vi "Conv_Meters_Feet.vi"(10 "Meters":dbl) -> (2 "Feet":dbl)   [LabVIEW 2019, in "PathExecution_Library.lvlib"]
doc: "Convert Feet to Meters"
uses:
  PathExecution_Library.lvlib
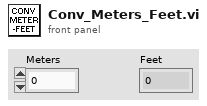
[diagram p1: front panel]
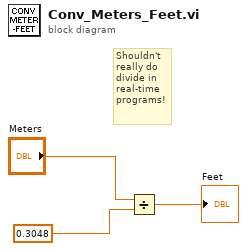
[diagram p0: block diagram]
diagram:
  # "Shouldn't\nreally do\ndivide in\nreal-time\nprograms!"
  n1 = Divide(x="Meters", y=0.3048) -> (x/y=→"Feet":dbl)
